vi "RunTestsFromCmdLine.vi"   [LabVIEW 2018]
uses:
  <vilib>/Wiresmith Technology/LabVIEW CLI/CLI Class/CLI.lvclass
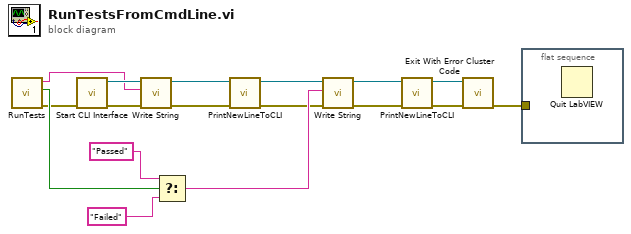
[diagram p0: block diagram]
diagram:
  n1 = call "RunTests.vi"() -> ("error out"=w10:errorcluster, "successful?"=w14:bool, "test details"=w16:string)  [unwired: 9 in]
  n2 = call <vilib>:"Start CLI Interface.vi"("error in (no error)"=w10) -> ("error out"=w15:errorcluster, "CLI out"=w17:refnum<class "CLI.lvclass">)  [unwired: 8 in, 1 out]
  n3 = call <vilib>:"Write String.vi"("error in (no error)"=w15, "Text to Write"=w16, "CLI in"=w17) -> ("error out"=w7:errorcluster, "CLI out"=w8:refnum<class "CLI.lvclass">)  [unwired: 7 in]
  n4 = Select(t="Passed", s=w14, f="Failed") -> (s? t:f=w11:string)
  n5 = call "PrintNewLineToCLI.vi"("error in (no error)"=w7, "CLI in"=w8) -> ("error out"=w6:errorcluster, "CLI out"=w5:refnum<class "CLI.lvclass">)  [unwired: 8 in]
  n6 = call <vilib>:"Write String.vi"("error in (no error)"=w6, "Text to Write"=w11, "CLI in"=w5) -> ("error out"=w1:errorcluster, "CLI out"=w2:refnum<class "CLI.lvclass">)  [unwired: 7 in]
  n7 = call "PrintNewLineToCLI.vi"("error in (no error)"=w1, "CLI in"=w2) -> ("error out"=w3:errorcluster, "CLI out"=w4:refnum<class "CLI.lvclass">)  [unwired: 8 in]
  n8 = call <vilib>:"Exit With Error Cluster Code.vi"("error in (no error)"=w3, "CLI in"=w4) -> ("error out"=w9:errorcluster)  [unwired: 9 in]
  n9 = flat-sequence {
    tunnel: w9 -> [_]
    frame #0 {
      n10 = Quit LabVIEW() -> ()  [unwired: 1 in]
    }
  }
